vi "Global communication.vi"() -> ()   [LabVIEW 2016]
panel:
  in  "Communication all":dbl[][](array[numeric])
  out "LC control":dbl[][](array[numeric])
  out "LC status":dbl[][](array[numeric])
  in  "Sources on/off":dbl[](array[numeric])
  in  "Switch communication":dbl[](array[numeric])
  in  "Gen LC communication":dbl[](array[numeric])
  in  "PV APF ave":dbl
  in  "PV APF 1 s":dbl[](array[numeric])
  in  "BESS APF ave":dbl
  in  "BESS APF 1 s":dbl[](array[numeric])
  in  "APF average":dbl[](array[numeric])
  in  "APF 1s":dbl[][](array[numeric])
  in  "PV LC communication":dbl[](array[numeric])
  in  "BESS LC communication":dbl[](array[numeric])
  in  "Status":dbl[](array[numeric])
  in  "RPF":dbl[](array[numeric])
  in  "Reserved15":dbl[](array[numeric])
  in  "Reserved14":dbl[](array[numeric])
  in  "Reserved13":dbl[](array[numeric])
  in  "MAG-C-R":dbl[](array[numeric])
  in  "MAG-C-L":dbl[](array[numeric])
  in  "MAG-B-R":dbl[](array[numeric])
  in  "MAG-B-L":dbl[](array[numeric])
  in  "MAG-A-R":dbl[](array[numeric])
  in  "MAG-A-L":dbl[](array[numeric])
  in  "FREQ-R":dbl[](array[numeric])
  in  "FREQ-L":dbl[](array[numeric])
  in  "APF":dbl[](array[numeric])
  in  "ANG-DIFF":dbl[](array[numeric])
  in  "Global communication":dbl[](array[numeric])
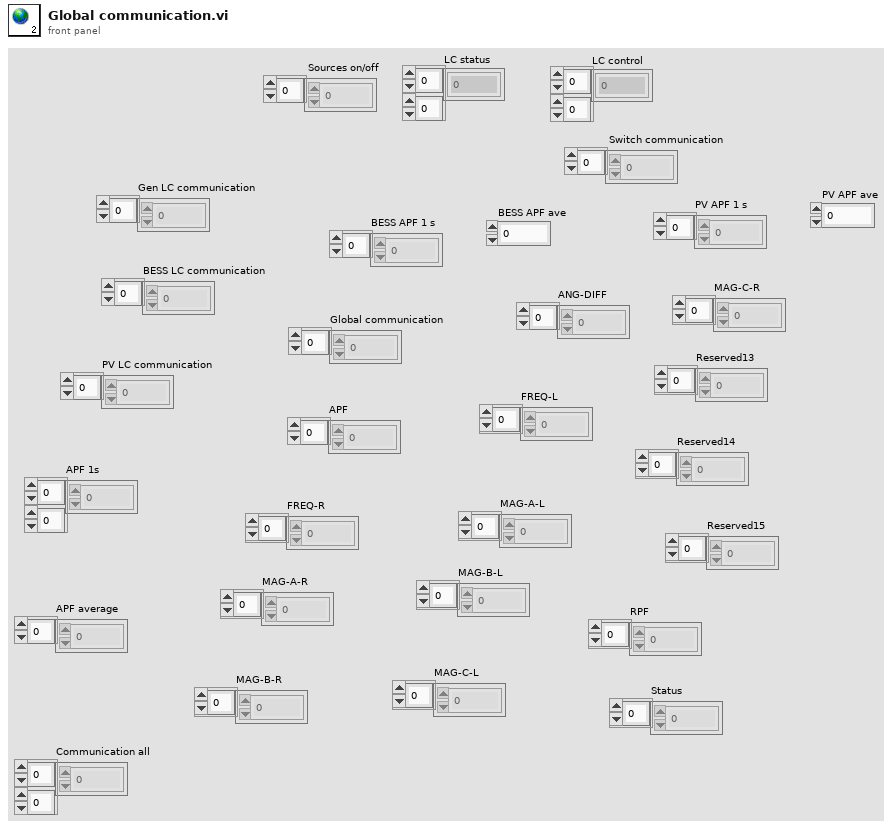
[diagram p1: front panel]
diagram:
